vi "LVJSON Unflatten.vi"(7 "Variant Type":variant, 8 "error in (no error)":errorcluster, 10 "Root Path ([]=Root)":string[](array[string]), 11 "Root Element in":T1) -> (0 "error out":errorcluster, 1 "Exists?":bool, 3 "Variant out":variant, 4 "Key":string)   [LabVIEW 2019, in "labview_json.lvlib"]
uses:
  labview_json.lvlib
  Element.ctl
  Element Type.ctl
  <vilib>/Utility/error.llb/Error Cluster From Error Code.vi
  <vilib>/ErrorRing/Error Ring.xnode
  <vilib>/Utility/Data Type/NI_Data Type.lvlib
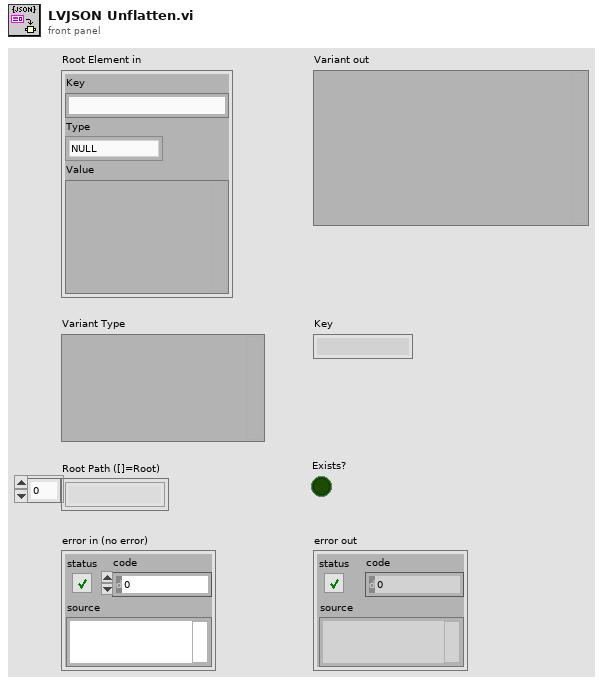
[diagram p1: front panel]
types:
  T1 = typedef "labview_json.lvlib/Element.ctl" = cluster{"Key":string, "Type":T2, "Value":variant}
  T2 = typedef "labview_json.lvlib/Element Type.ctl" = enum8{"NULL", "BOOL", "INT", "UINT", "FLOAT", "STRING", "ARRAY", "OBJECT", "SKIP"}
  T3 = typedef "NI_Data Type.lvlib/Data Type.ctl" = enum8{"Invalid Type", "Void", "I8", "I16", "I32", "I64", "U8", "U16", "U32", "U64", "Single Float", "Double Float", "Extended Float", "Single Complex", "Double Complex", "Extended Complex", "Enum U8", "Enum U16", "Enum U32", "Enum U64", "Single Float With Unit", "Double Float With Unit", "Extended Float With Unit", "Single Complex with Unit", "Double Complex with Unit", "Extended Complex with Unit", "Boolean", "String", "Path", "Picture", "Tag", "Array", "Cluster", "Variant", "LV Variant", "Waveform", "Timestamp", "Digital Waveform", "Digital Data", "ExpressData", "Refnum", "External Data", "VI", "Poly VI", "LabVIEW Class Instance", "Fixed Point", "Set Collection", "Map Collection"}
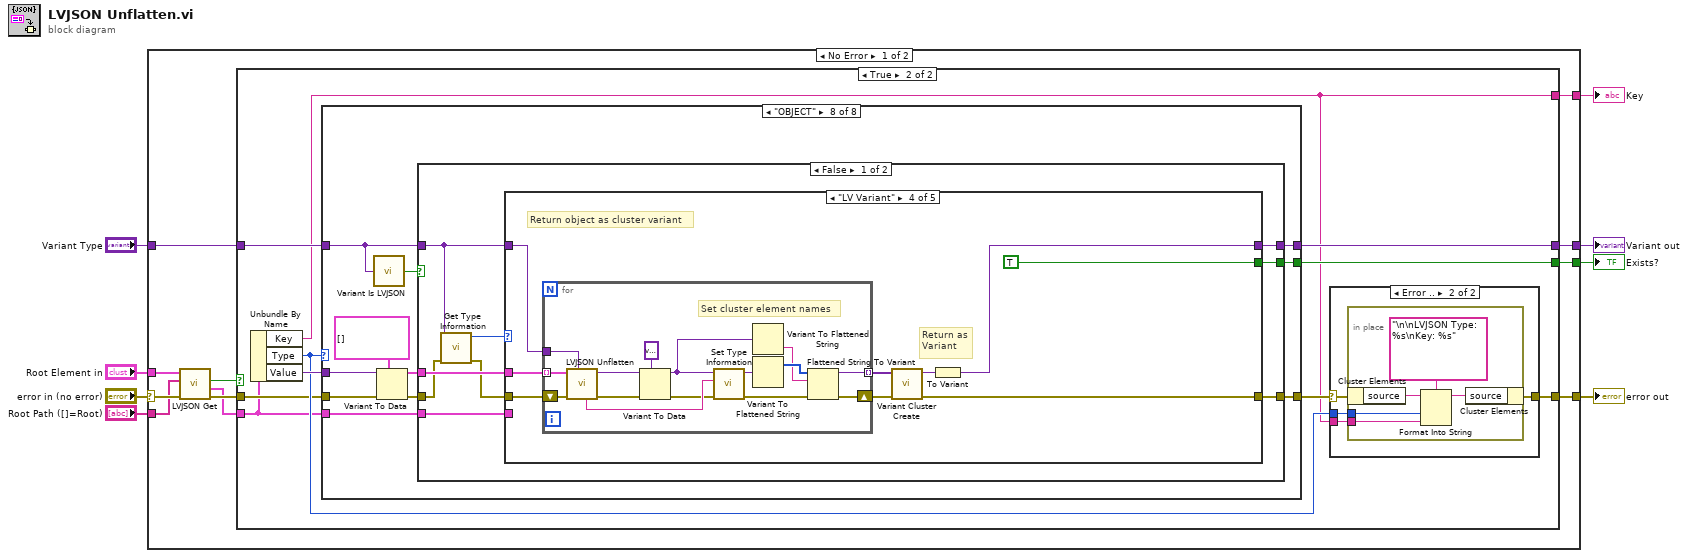
[diagram p0: block diagram]
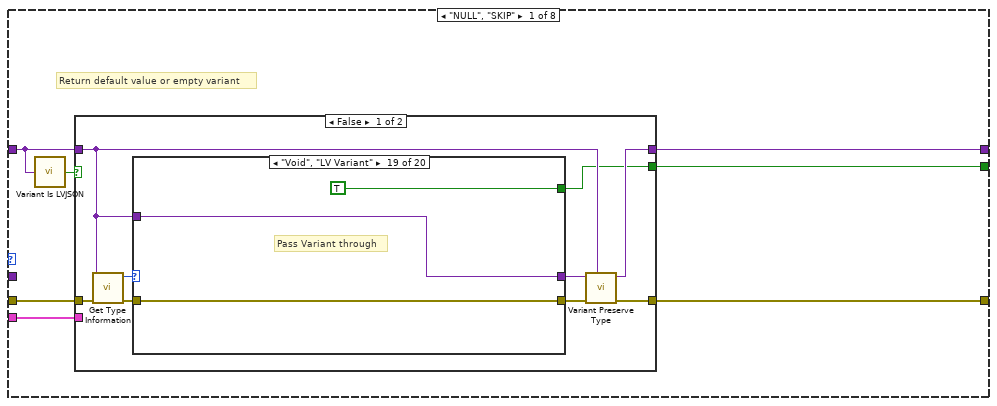
[diagram p3: hidden frame]
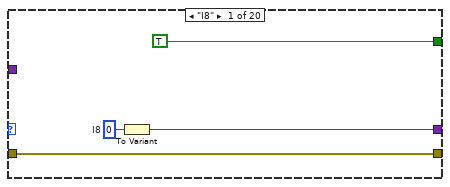
[diagram p4: hidden frame]
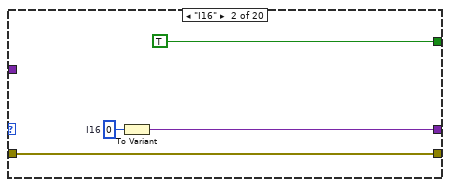
[diagram p5: hidden frame]
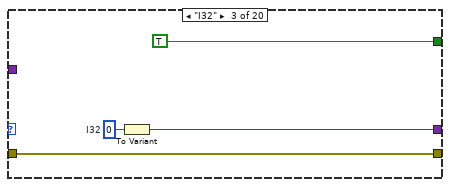
[diagram p6: hidden frame]
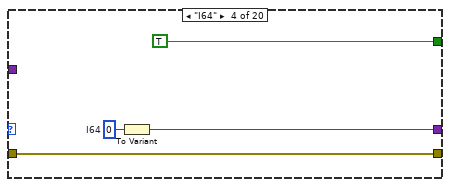
[diagram p7: hidden frame]
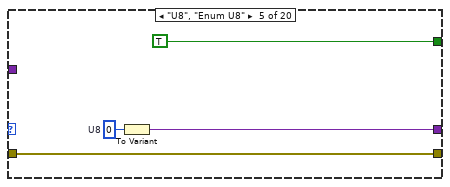
[diagram p8: hidden frame]
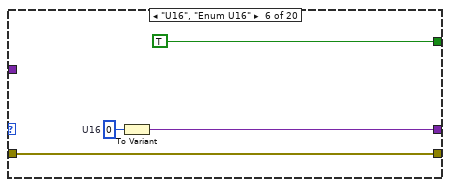
[diagram p9: hidden frame]
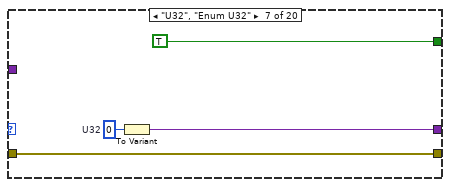
[diagram p10: hidden frame]
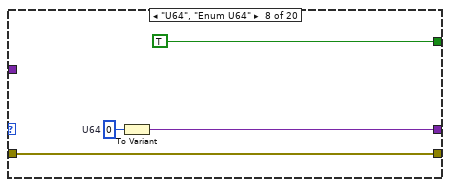
[diagram p11: hidden frame]
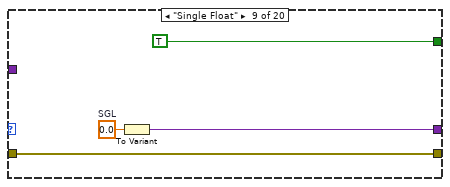
[diagram p12: hidden frame]
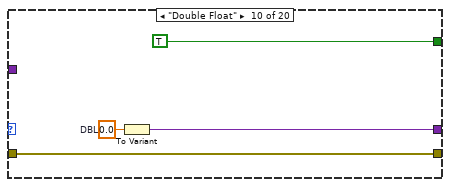
[diagram p13: hidden frame]
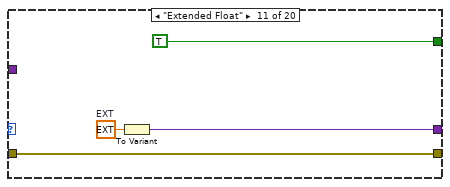
[diagram p14: hidden frame]
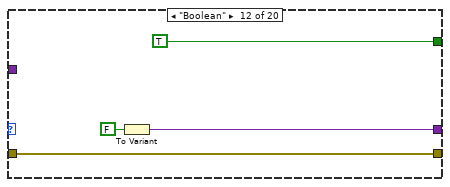
[diagram p15: hidden frame]
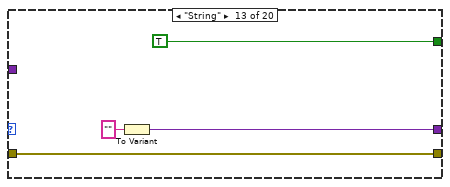
[diagram p16: hidden frame]
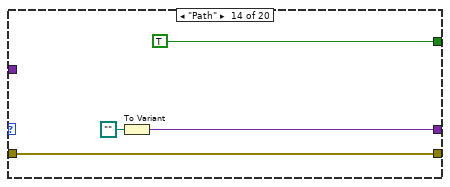
[diagram p17: hidden frame]
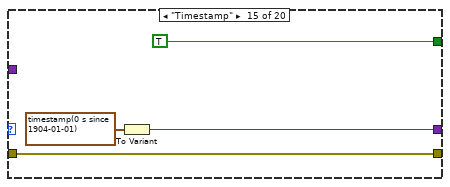
[diagram p18: hidden frame]
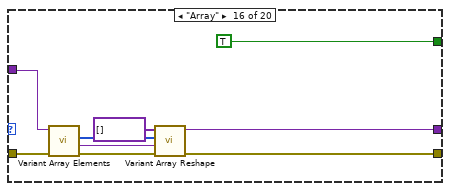
[diagram p19: hidden frame]
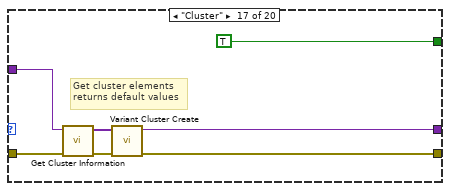
[diagram p20: hidden frame]
diagram:
  n1 = case shown="No Error" "error in (no error)" {
    selector: "error in (no error)" -> [w14 w1004]
    tunnel: "Root Element in" -> [w12 _]
    tunnel: [w19 w1004] -> w8
    tunnel: "Variant Type" -> [w18 w1003]
    tunnel: [w15 _] -> w4
    tunnel: [w17 w1003] -> w3
    tunnel: [w16 _] -> w2
    tunnel: "Root Path ([]=Root)" -> [w11 _]
    frame No Error {
      n2 = call "LVJSON Get.vi"("error in (no error)"=w14, "Root Path ([]=Root)"=w11, "Root Element in"=w12) -> ("error out"=w13:errorcluster, "Element out"=w10:T1, "Exists?"=w9:bool)  [unwired: 5 in, 1 out]
      n3 = case shown="True" w9 {
        tunnel: [w21 w31] -> w19
        tunnel: w18 -> [w20 w30]
        tunnel: [w20 w29] -> w17
        tunnel: [_ w27] -> w16
        tunnel: [_ w24] -> w15
        tunnel: w13 -> [w21 w23]
        tunnel: w10 -> [_ w22]
        frame False {
        }
        frame True {
          n4 = Unbundle By Name(w22) -> ("Key"=w24:string, "Type"=w25:T2, "Value"=w26:variant)
          n5 = case shown="\"OBJECT\"" w25 {
            tunnel: [w38 w160 w213 w317 w421 w525 w664 w834] -> w29
            tunnel: w23 -> [w32 w156 w208 w312 w416 w520 w668 w838]
            tunnel: w30 -> [w35 w150 w205 w309 w413 w517 w661 w830]
            tunnel: w22 -> [w33 w152 w203 w307 w411 w515 w660 w832]
            tunnel: w26 -> [_ w155 w207 w311 w415 w519 w667 w837]
            tunnel: [w37 w159 w212 w316 w420 w524 w663 w833] -> w28
            tunnel: [w36 w154 w206 w310 w414 w518 w662 w831] -> w27
            frame "NULL", "SKIP" {
              # "Return default value or empty variant"
              n6 = call "Variant Is LVJSON.vi"("Variant"=w35) -> ("Is LVJSON?"=w34:bool)
              n7 = case shown="False" w34 {
                tunnel: [w47 w148] -> w38
                tunnel: [w46 w146] -> w37
                tunnel: [w39 TRUE] -> w36
                tunnel: w32 -> [w41 w146]
                tunnel: w35 -> [w40 _]
                tunnel: w33 -> [_ w149]
                frame False {
                  n8 = call <vilib>:"Get Type Information.vi"("error in (no error)"=w41, "variant"=w40) -> ("error out"=w42:errorcluster, "type"=w43:T3)  [unwired: 5 in, 3 out]
                  n9 = case shown="\"Void\", \"LV Variant\"" w43 {
                    selector: w43 -> [_ _ _ _ _ _ _ _ _ _ _ _ _ _ _ _ _ _ _ w133]
                    tunnel: [w51 w55 w59 w63 w67 w71 w75 w79 w83 w87 w91 w95 w99 w103 w107 w112 w122 w127 w130 w132] -> w45
                    tunnel: w42 -> [w51 w55 w59 w63 w67 w71 w75 w79 w83 w87 w91 w95 w99 w103 w107 w110 w121 w127 w130 w137]
                    tunnel: [w50 w54 w58 w62 w66 w70 w74 w78 w82 w86 w90 w94 w98 w102 w106 w111 w118 w126 w128 w138] -> w44
                    tunnel: w40 -> [_ _ _ _ _ _ _ _ _ _ _ _ _ _ _ w109 w120 _ w128 w138]
                    tunnel: [TRUE TRUE TRUE TRUE TRUE TRUE TRUE TRUE TRUE TRUE TRUE TRUE TRUE TRUE TRUE TRUE TRUE TRUE TRUE FALSE] -> w39
                    frame "I8" {
                      w49 = i8 0  # I8
                      n10 = To Variant(anything=w49) -> (Variant=w50:variant)
                    }
                    frame "I16" {
                      w53 = i16 0  # I16
                      n11 = To Variant(anything=w53) -> (Variant=w54:variant)
                    }
                    frame "I32" {
                      w57 = 0  # I32
                      n12 = To Variant(anything=w57) -> (Variant=w58:variant)
                    }
                    frame "I64" {
                      w61 = i64 0  # I64
                      n13 = To Variant(anything=w61) -> (Variant=w62:variant)
                    }
                    frame "U8", "Enum U8" {
                      w65 = u8 0  # U8
                      n14 = To Variant(anything=w65) -> (Variant=w66:variant)
                    }
                    frame "U16", "Enum U16" {
                      w69 = u16 0  # U16
                      n15 = To Variant(anything=w69) -> (Variant=w70:variant)
                    }
                    frame "U32", "Enum U32" {
                      w73 = u32 0  # U32
                      n16 = To Variant(anything=w73) -> (Variant=w74:variant)
                    }
                    frame "U64", "Enum U64" {
                      w77 = u64 0  # U64
                      n17 = To Variant(anything=w77) -> (Variant=w78:variant)
                    }
                    frame "Single Float" {
                      w81 = sgl 0.0  # SGL
                      n18 = To Variant(anything=w81) -> (Variant=w82:variant)
                    }
                    frame "Double Float" {
                      w85 = 0.0  # DBL
                      n19 = To Variant(anything=w85) -> (Variant=w86:variant)
                    }
                    frame "Extended Float" {
                      w89 = ext 0.0  # EXT
                      n20 = To Variant(anything=w89) -> (Variant=w90:variant)
                    }
                    frame "Boolean" {
                      n21 = To Variant(anything=FALSE) -> (Variant=w94:variant)
                    }
                    frame "String" {
                      n22 = To Variant(anything="") -> (Variant=w98:variant)
                    }
                    frame "Path" {
                      n23 = To Variant(anything=path "" ("Not A Path Constant")) -> (Variant=w102:variant)
                    }
                    frame "Timestamp" {
                      n24 = To Variant(anything=timestamp(0 s since 1904-01-01)) -> (Variant=w106:variant)
                    }
                    frame "Array" {
                      n25 = call "Variant Array Elements.vi"("error in (no error)"=w110, "N Dim Array"=w109) -> ("error out"=w113:errorcluster, "Element Type"=w114:variant, "Sizes"=w115:i32[])  [unwired: 6 in, 1 out]
                      n26 = call "Variant Array Reshape.vi"("error in (no error)"=w113, "Default Element Type"=w114, "Sizes"=w115, "Elements"=variant[] []) -> ("error out"=w112:errorcluster, "N Dim Array"=w111:variant)  [unwired: 6 in]
                    }
                    frame "Cluster" {
                      # "Get cluster elements\nreturns default values"
                      n27 = call <vilib>:"Get Cluster Information.vi"("error in (no error)"=w121, "variant"=w120) -> ("error out"=w117:errorcluster, "cluster elements"=w119:variant[])  [unwired: 8 in]
                      n28 = call "Variant Cluster Create.vi"("error in (no error)"=w117, "Elements"=w119) -> ("error out"=w122:errorcluster, "Cluster"=w118:variant)  [unwired: 8 in]
                    }
                    frame "Waveform" {
                      n29 = To Variant(anything=waveform(dbl) {"t0"=timestamp(0 s since 1904-01-01), "dt"=0.0, "Y"=[]} ("Waveform")) -> (Variant=w126:variant)
                    }
                    frame "Void", "LV Variant" {
                      # "Pass Variant through"
                    }
                    frame Default {
                      n30 = Format Into String(format string="%s", w133) -> (resulting string=w135:string)  [unwired: 2 in, 1 out]
                      n31 = xnode "Error Ring"("parameter 0"=w135) -> ("error out"=w131:errorcluster)
                      n32 = Merge Errors(w137, w131) -> (w132:errorcluster)
                    }
                  }
                  n33 = call "Variant Preserve Type.vi"("Variant Type"=w40, "error in (no error)"=w45, "Variant in"=w44) -> ("error out"=w46:errorcluster, "Variant out"=w47:variant)  [unwired: 7 in]
                }
                frame True {
                  # "Return element as LVJSON object"
                  n34 = To Variant(anything=w149) -> (Variant=w148:variant)
                }
              }
            }
            frame "BOOL" {
              # "Return boolean"
              n35 = Variant To Data(error in=w156, type=FALSE, Variant=w155) -> (data=w158:bool, error out=w151:errorcluster)
              n36 = call "Variant Is LVJSON.vi"("Variant"=w150) -> ("Is LVJSON?"=w153:bool)
              n37 = case shown="False" w153 {
                tunnel: [w170 w201] -> w160
                tunnel: [w169 w199] -> w159
                tunnel: w158 -> [w168 _]
                tunnel: [w162 TRUE] -> w154
                tunnel: w151 -> [w165 w199]
                tunnel: w150 -> [w161 _]
                tunnel: w152 -> [_ w202]
                frame False {
                  n38 = call <vilib>:"Get Type Information.vi"("error in (no error)"=w165, "variant"=w161) -> ("error out"=w163:errorcluster, "type"=w166:T3)  [unwired: 5 in, 3 out]
                  n39 = case shown="\"Void\"" w166 {
                    selector: w166 -> [w171 _ _ _]
                    tunnel: w168 -> [_ w189 w193 w197]
                    tunnel: [w177 w188 w191 w195] -> w167
                    tunnel: [w173 w187 w190 w196] -> w164
                    tunnel: w163 -> [w178 w187 w190 w196]
                    tunnel: [FALSE TRUE TRUE TRUE] -> w162
                    tunnel: w161 -> [w177 _ _ _]
                    frame Default {
                      n40 = Format Into String(format string="%s", w171) -> (resulting string=w175:string)  [unwired: 2 in, 1 out]
                      n41 = xnode "Error Ring"("parameter 0"=w175) -> ("error out"=w172:errorcluster)
                      n42 = Merge Errors(w178, w172) -> (w173:errorcluster)
                    }
                    frame "Boolean" {
                      n43 = To Variant(anything=w189) -> (Variant=w188:variant)
                    }
                    frame "LV Variant" {
                      n44 = To Variant(anything=w193) -> (Variant=w192:variant)
                      n45 = To Variant(anything=w192) -> (Variant=w191:variant)
                    }
                    frame "Void" {
                      n46 = To Variant(anything=w197) -> (Variant=w195:variant)
                    }
                  }
                  n47 = call "Variant Preserve Type.vi"("Variant Type"=w161, "error in (no error)"=w164, "Variant in"=w167) -> ("error out"=w169:errorcluster, "Variant out"=w170:variant)  [unwired: 7 in]
                }
                frame True {
                  # "Return element as LVJSON object"
                  n48 = To Variant(anything=w202) -> (Variant=w201:variant)
                }
              }
            }
            frame "INT" {
              w211 = i64 0  # I64
              # "Return int as int, uint, float or variant"
              n49 = call "Variant Is LVJSON.vi"("Variant"=w205) -> ("Is LVJSON?"=w204:bool)
              n50 = Variant To Data(error in=w208, type=w211, Variant=w207) -> (data=w209:i64, error out=w210:errorcluster)
              n51 = case shown="False" w204 {
                tunnel: [w223 w305] -> w213
                tunnel: [w222 w303] -> w212
                tunnel: w210 -> [w217 w303]
                tunnel: w209 -> [w221 _]
                tunnel: [w214 TRUE] -> w206
                tunnel: w205 -> [w215 _]
                tunnel: w203 -> [_ w306]
                frame False {
                  n52 = call <vilib>:"Get Type Information.vi"("error in (no error)"=w217, "variant"=w215) -> ("error out"=w218:errorcluster, "type"=w216:T3)  [unwired: 5 in, 3 out]
                  n53 = case shown="\"Void\"" w216 {
                    selector: w216 -> [w228 _ _ _ _ _ _ _ _ _ _ _ _ _]
                    tunnel: [w227 w242 w247 w252 w257 w262 w267 w272 w277 w282 w287 w292 w298 w302] -> w220
                    tunnel: w218 -> [w231 w242 w247 w252 w257 w262 w267 w272 w277 w282 w287 w292 w298 w302]
                    tunnel: [w225 w240 w245 w250 w255 w260 w265 w270 w275 w280 w285 w290 w296 w299] -> w219
                    tunnel: w221 -> [_ w243 w248 w253 w258 w263 w268 w273 w278 w283 w288 w293 w297 w301]
                    tunnel: w215 -> [w225 _ _ _ _ _ _ _ _ _ _ _ _ _]
                    tunnel: [FALSE TRUE TRUE TRUE TRUE TRUE TRUE TRUE TRUE TRUE TRUE TRUE TRUE TRUE] -> w214
                    frame Default {
                      n54 = Format Into String(format string="%s", w228) -> (resulting string=w230:string)  [unwired: 2 in, 1 out]
                      n55 = xnode "Error Ring"("parameter 0"=w230) -> ("error out"=w226:errorcluster)
                      n56 = Merge Errors(w231, w226) -> (w227:errorcluster)
                    }
                    frame "I8" {
                      n57 = To Byte Integer(number=w243) -> (8bit integer=w241:i8)
                      n58 = To Variant(anything=w241) -> (Variant=w240:variant)
                    }
                    frame "I16" {
                      n59 = To Word Integer(number=w248) -> (16bit integer=w246:i16)
                      n60 = To Variant(anything=w246) -> (Variant=w245:variant)
                    }
                    frame "I32" {
                      n61 = To Long Integer(number=w253) -> (32bit integer=w251:i32)
                      n62 = To Variant(anything=w251) -> (Variant=w250:variant)
                    }
                    frame "I64" {
                      n63 = To Quad Integer(1:w258) -> (0:w256:i64)
                      n64 = To Variant(anything=w256) -> (Variant=w255:variant)
                    }
                    frame "U8", "Enum U8" {
                      n65 = To Unsigned Byte Integer(number=w263) -> (unsigned 8bit integer=w261:u8)
                      n66 = To Variant(anything=w261) -> (Variant=w260:variant)
                    }
                    frame "U16", "Enum U16" {
                      n67 = To Unsigned Word Integer(number=w268) -> (unsigned 16bit integer=w266:u16)
                      n68 = To Variant(anything=w266) -> (Variant=w265:variant)
                    }
                    frame "U32", "Enum U32" {
                      n69 = To Unsigned Long Integer(number=w273) -> (unsigned 32bit integer=w271:u32)
                      n70 = To Variant(anything=w271) -> (Variant=w270:variant)
                    }
                    frame "U64", "Enum U64" {
                      n71 = To Unsigned Quad Integer(1:w278) -> (0:w276:u64)
                      n72 = To Variant(anything=w276) -> (Variant=w275:variant)
                    }
                    frame "Single Float" {
                      n73 = To Single Precision Float(number=w283) -> (single precision float=w281:sgl)
                      n74 = To Variant(anything=w281) -> (Variant=w280:variant)
                    }
                    frame "Double Float" {
                      n75 = To Double Precision Float(number=w288) -> (double precision float=w286:dbl)
                      n76 = To Variant(anything=w286) -> (Variant=w285:variant)
                    }
                    frame "Extended Float" {
                      n77 = To Extended Precision Float(1:w293) -> (0:w291:ext)
                      n78 = To Variant(anything=w291) -> (Variant=w290:variant)
                    }
                    frame "LV Variant" {
                      n79 = To Variant(anything=w297) -> (Variant=w295:variant)
                      n80 = To Variant(anything=w295) -> (Variant=w296:variant)
                    }
                    frame "Void" {
                      n81 = To Variant(anything=w301) -> (Variant=w299:variant)
                    }
                  }
                  n82 = call "Variant Preserve Type.vi"("Variant Type"=w215, "error in (no error)"=w220, "Variant in"=w219) -> ("error out"=w222:errorcluster, "Variant out"=w223:variant)  [unwired: 7 in]
                }
                frame True {
                  # "Return element as LVJSON object"
                  n83 = To Variant(anything=w306) -> (Variant=w305:variant)
                }
              }
            }
            frame "UINT" {
              w315 = u64 0  # U64
              # "Return int as int, uint, float or variant"
              n84 = call "Variant Is LVJSON.vi"("Variant"=w309) -> ("Is LVJSON?"=w308:bool)
              n85 = Variant To Data(error in=w312, type=w315, Variant=w311) -> (data=w313:u64, error out=w314:errorcluster)
              n86 = case shown="False" w308 {
                tunnel: [w327 w409] -> w317
                tunnel: [w326 w407] -> w316
                tunnel: w314 -> [w321 w407]
                tunnel: w313 -> [w325 _]
                tunnel: [w318 TRUE] -> w310
                tunnel: w309 -> [w319 _]
                tunnel: w307 -> [_ w410]
                frame False {
                  n87 = call <vilib>:"Get Type Information.vi"("error in (no error)"=w321, "variant"=w319) -> ("error out"=w322:errorcluster, "type"=w320:T3)  [unwired: 5 in, 3 out]
                  n88 = case shown="\"Void\"" w320 {
                    selector: w320 -> [w332 _ _ _ _ _ _ _ _ _ _ _ _ _]
                    tunnel: [w331 w346 w351 w356 w361 w366 w371 w376 w381 w386 w391 w396 w402 w406] -> w324
                    tunnel: w322 -> [w335 w346 w351 w356 w361 w366 w371 w376 w381 w386 w391 w396 w402 w406]
                    tunnel: [w329 w344 w349 w354 w359 w364 w369 w374 w379 w384 w389 w394 w400 w403] -> w323
                    tunnel: w325 -> [_ w347 w352 w357 w362 w367 w372 w377 w382 w387 w392 w397 w401 w405]
                    tunnel: w319 -> [w329 _ _ _ _ _ _ _ _ _ _ _ _ _]
                    tunnel: [FALSE TRUE TRUE TRUE TRUE TRUE TRUE TRUE TRUE TRUE TRUE TRUE TRUE TRUE] -> w318
                    frame Default {
                      n89 = Format Into String(format string="%s", w332) -> (resulting string=w334:string)  [unwired: 2 in, 1 out]
                      n90 = xnode "Error Ring"("parameter 0"=w334) -> ("error out"=w330:errorcluster)
                      n91 = Merge Errors(w335, w330) -> (w331:errorcluster)
                    }
                    frame "I8" {
                      n92 = To Byte Integer(number=w347) -> (8bit integer=w345:i8)
                      n93 = To Variant(anything=w345) -> (Variant=w344:variant)
                    }
                    frame "I16" {
                      n94 = To Word Integer(number=w352) -> (16bit integer=w350:i16)
                      n95 = To Variant(anything=w350) -> (Variant=w349:variant)
                    }
                    frame "I32" {
                      n96 = To Long Integer(number=w357) -> (32bit integer=w355:i32)
                      n97 = To Variant(anything=w355) -> (Variant=w354:variant)
                    }
                    frame "I64" {
                      n98 = To Quad Integer(1:w362) -> (0:w360:i64)
                      n99 = To Variant(anything=w360) -> (Variant=w359:variant)
                    }
                    frame "U8", "Enum U8" {
                      n100 = To Unsigned Byte Integer(number=w367) -> (unsigned 8bit integer=w365:u8)
                      n101 = To Variant(anything=w365) -> (Variant=w364:variant)
                    }
                    frame "U16", "Enum U16" {
                      n102 = To Unsigned Word Integer(number=w372) -> (unsigned 16bit integer=w370:u16)
                      n103 = To Variant(anything=w370) -> (Variant=w369:variant)
                    }
                    frame "U32", "Enum U32" {
                      n104 = To Unsigned Long Integer(number=w377) -> (unsigned 32bit integer=w375:u32)
                      n105 = To Variant(anything=w375) -> (Variant=w374:variant)
                    }
                    frame "U64", "Enum U64" {
                      n106 = To Unsigned Quad Integer(1:w382) -> (0:w380:u64)
                      n107 = To Variant(anything=w380) -> (Variant=w379:variant)
                    }
                    frame "Single Float" {
                      n108 = To Single Precision Float(number=w387) -> (single precision float=w385:sgl)
                      n109 = To Variant(anything=w385) -> (Variant=w384:variant)
                    }
                    frame "Double Float" {
                      n110 = To Double Precision Float(number=w392) -> (double precision float=w390:dbl)
                      n111 = To Variant(anything=w390) -> (Variant=w389:variant)
                    }
                    frame "Extended Float" {
                      n112 = To Extended Precision Float(1:w397) -> (0:w395:ext)
                      n113 = To Variant(anything=w395) -> (Variant=w394:variant)
                    }
                    frame "LV Variant" {
                      n114 = To Variant(anything=w401) -> (Variant=w399:variant)
                      n115 = To Variant(anything=w399) -> (Variant=w400:variant)
                    }
                    frame "Void" {
                      n116 = To Variant(anything=w405) -> (Variant=w403:variant)
                    }
                  }
                  n117 = call "Variant Preserve Type.vi"("Variant Type"=w319, "error in (no error)"=w324, "Variant in"=w323) -> ("error out"=w326:errorcluster, "Variant out"=w327:variant)  [unwired: 7 in]
                }
                frame True {
                  # "Return element as LVJSON object"
                  n118 = To Variant(anything=w410) -> (Variant=w409:variant)
                }
              }
            }
            frame "FLOAT" {
              w419 = 0.0  # DBL
              # "Return int as int, uint, float or variant"
              n119 = call "Variant Is LVJSON.vi"("Variant"=w413) -> ("Is LVJSON?"=w412:bool)
              n120 = Variant To Data(error in=w416, type=w419, Variant=w415) -> (data=w417:dbl, error out=w418:errorcluster)
              n121 = case shown="False" w412 {
                tunnel: [w431 w513] -> w421
                tunnel: [w430 w511] -> w420
                tunnel: w418 -> [w425 w511]
                tunnel: w417 -> [w429 _]
                tunnel: [w422 TRUE] -> w414
                tunnel: w413 -> [w423 _]
                tunnel: w411 -> [_ w514]
                frame False {
                  n122 = call <vilib>:"Get Type Information.vi"("error in (no error)"=w425, "variant"=w423) -> ("error out"=w426:errorcluster, "type"=w424:T3)  [unwired: 5 in, 3 out]
                  n123 = case shown="\"Void\"" w424 {
                    selector: w424 -> [w436 _ _ _ _ _ _ _ _ _ _ _ _ _]
                    tunnel: [w435 w450 w455 w460 w465 w470 w475 w480 w485 w490 w495 w500 w506 w510] -> w428
                    tunnel: w426 -> [w439 w450 w455 w460 w465 w470 w475 w480 w485 w490 w495 w500 w506 w510]
                    tunnel: [w433 w448 w453 w458 w463 w468 w473 w478 w483 w488 w493 w498 w504 w507] -> w427
                    tunnel: w429 -> [_ w451 w456 w461 w466 w471 w476 w481 w486 w491 w496 w501 w505 w509]
                    tunnel: w423 -> [w433 _ _ _ _ _ _ _ _ _ _ _ _ _]
                    tunnel: [FALSE TRUE TRUE TRUE TRUE TRUE TRUE TRUE TRUE TRUE TRUE TRUE TRUE TRUE] -> w422
                    frame Default {
                      n124 = Format Into String(format string="%s", w436) -> (resulting string=w438:string)  [unwired: 2 in, 1 out]
                      n125 = xnode "Error Ring"("parameter 0"=w438) -> ("error out"=w434:errorcluster)
                      n126 = Merge Errors(w439, w434) -> (w435:errorcluster)
                    }
                    frame "I8" {
                      n127 = To Byte Integer(number=w451) -> (8bit integer=w449:i8)
                      n128 = To Variant(anything=w449) -> (Variant=w448:variant)
                    }
                    frame "I16" {
                      n129 = To Word Integer(number=w456) -> (16bit integer=w454:i16)
                      n130 = To Variant(anything=w454) -> (Variant=w453:variant)
                    }
                    frame "I32" {
                      n131 = To Long Integer(number=w461) -> (32bit integer=w459:i32)
                      n132 = To Variant(anything=w459) -> (Variant=w458:variant)
                    }
                    frame "I64" {
                      n133 = To Quad Integer(1:w466) -> (0:w464:i64)
                      n134 = To Variant(anything=w464) -> (Variant=w463:variant)
                    }
                    frame "U8", "Enum U8" {
                      n135 = To Unsigned Byte Integer(number=w471) -> (unsigned 8bit integer=w469:u8)
                      n136 = To Variant(anything=w469) -> (Variant=w468:variant)
                    }
                    frame "U16", "Enum U16" {
                      n137 = To Unsigned Word Integer(number=w476) -> (unsigned 16bit integer=w474:u16)
                      n138 = To Variant(anything=w474) -> (Variant=w473:variant)
                    }
                    frame "U32", "Enum U32" {
                      n139 = To Unsigned Long Integer(number=w481) -> (unsigned 32bit integer=w479:u32)
                      n140 = To Variant(anything=w479) -> (Variant=w478:variant)
                    }
                    frame "U64", "Enum U64" {
                      n141 = To Unsigned Quad Integer(1:w486) -> (0:w484:u64)
                      n142 = To Variant(anything=w484) -> (Variant=w483:variant)
                    }
                    frame "Single Float" {
                      n143 = To Single Precision Float(number=w491) -> (single precision float=w489:sgl)
                      n144 = To Variant(anything=w489) -> (Variant=w488:variant)
                    }
                    frame "Double Float" {
                      n145 = To Double Precision Float(number=w496) -> (double precision float=w494:dbl)
                      n146 = To Variant(anything=w494) -> (Variant=w493:variant)
                    }
                    frame "Extended Float" {
                      n147 = To Extended Precision Float(1:w501) -> (0:w499:ext)
                      n148 = To Variant(anything=w499) -> (Variant=w498:variant)
                    }
                    frame "LV Variant" {
                      n149 = To Variant(anything=w505) -> (Variant=w503:variant)
                      n150 = To Variant(anything=w503) -> (Variant=w504:variant)
                    }
                    frame "Void" {
                      n151 = To Variant(anything=w509) -> (Variant=w507:variant)
                    }
                  }
                  n152 = call "Variant Preserve Type.vi"("Variant Type"=w423, "error in (no error)"=w428, "Variant in"=w427) -> ("error out"=w430:errorcluster, "Variant out"=w431:variant)  [unwired: 7 in]
                }
                frame True {
                  # "Return element as LVJSON object"
                  n153 = To Variant(anything=w514) -> (Variant=w513:variant)
                }
              }
            }
            frame "STRING" {
              # "Return string as string, enum, path, timestamp or variant"
              n154 = Variant To Data(error in=w520, type="", Variant=w519) -> (data=w522:string, error out=w523:errorcluster)
              n155 = call "Variant Is LVJSON.vi"("Variant"=w517) -> ("Is LVJSON?"=w516:bool)
              n156 = case shown="False" w516 {
                tunnel: [w535 w657] -> w525
                tunnel: [w534 w655] -> w524
                tunnel: w523 -> [w528 w655]
                tunnel: w522 -> [w533 _]
                tunnel: w517 -> [w530 _]
                tunnel: [w526 TRUE] -> w518
                tunnel: w515 -> [_ w658]
                frame False {
                  n157 = call <vilib>:"Get Type Information.vi"("error in (no error)"=w528, "variant"=w530) -> ("error out"=w529:errorcluster, "type"=w527:T3)  [unwired: 5 in, 3 out]
                  n158 = case shown="\"Void\"" w527 {
                    selector: w527 -> [w538 _ _ _ _ _ _ _ _]
                    tunnel: [w537 w553 w580 w607 w635 w640 w645 w649 w654] -> w531
                    tunnel: w529 -> [w543 w557 w584 w611 w635 w640 w645 w649 w654]
                    tunnel: [w542 w560 w587 w614 w634 w639 w643 w646 w653] -> w532
                    tunnel: w533 -> [_ w556 w583 w610 w633 w638 w644 w648 w652]
                    tunnel: w530 -> [w542 w559 w586 w613 _ _ _ _ _]
                    tunnel: [FALSE w552 w579 w606 TRUE TRUE TRUE TRUE TRUE] -> w526
                    frame Default {
                      n159 = Format Into String(format string="%s", w538) -> (resulting string=w540:string)  [unwired: 2 in, 1 out]
                      n160 = xnode "Error Ring"("parameter 0"=w540) -> ("error out"=w536:errorcluster)
                      n161 = Merge Errors(w543, w536) -> (w537:errorcluster)
                    }
                    frame "Enum U8" {
                      n162 = call <vilib>:"Get Numeric Information.vi"("error in (no error)"=w557, "variant"=w559) -> ("error out"=w554:errorcluster, "enum names"=w558:string[])  [unwired: 6 in, 2 out]
                      n163 = Search 1D Array(1D array=w558, element=w556) -> (index of element=w555:i32)  [unwired: 1 in]
                      n164 = case shown="..-1" w555 {
                        selector: w555 -> [w562 _]
                        tunnel: w556 -> [_ w570]
                        tunnel: w554 -> [w563 w569]
                        tunnel: [w563 w566] -> w553
                        tunnel: [TRUE FALSE] -> w552
                        tunnel: [w564 u8 0] -> w551
                        frame 0.. {
                          n165 = To Unsigned Byte Integer(number=w562) -> (unsigned 8bit integer=w564:u8)
                        }
                        frame ..-1 {
                          n166 = xnode "Error Ring"("parameter 0"=w570) -> ("error out"=w565:errorcluster)
                          n167 = Merge Errors(w569, w565) -> (w566:errorcluster)
                        }
                      }
                      n168 = To Variant(anything=w551) -> (Variant=w560:variant)
                    }
                    frame "Enum U16" {
                      n169 = call <vilib>:"Get Numeric Information.vi"("error in (no error)"=w584, "variant"=w586) -> ("error out"=w581:errorcluster, "enum names"=w585:string[])  [unwired: 6 in, 2 out]
                      n170 = Search 1D Array(1D array=w585, element=w583) -> (index of element=w582:i32)  [unwired: 1 in]
                      n171 = case shown="..-1" w582 {
                        selector: w582 -> [w589 _]
                        tunnel: w583 -> [_ w597]
                        tunnel: w581 -> [w590 w596]
                        tunnel: [w590 w593] -> w580
                        tunnel: [TRUE FALSE] -> w579
                        tunnel: [w591 u16 0] -> w578
                        frame 0.. {
                          n172 = To Unsigned Word Integer(number=w589) -> (unsigned 16bit integer=w591:u16)
                        }
                        frame ..-1 {
                          n173 = xnode "Error Ring"("parameter 0"=w597) -> ("error out"=w592:errorcluster)
                          n174 = Merge Errors(w596, w592) -> (w593:errorcluster)
                        }
                      }
                      n175 = To Variant(anything=w578) -> (Variant=w587:variant)
                    }
                    frame "Enum U32" {
                      n176 = call <vilib>:"Get Numeric Information.vi"("error in (no error)"=w611, "variant"=w613) -> ("error out"=w608:errorcluster, "enum names"=w612:string[])  [unwired: 6 in, 2 out]
                      n177 = Search 1D Array(1D array=w612, element=w610) -> (index of element=w609:i32)  [unwired: 1 in]
                      n178 = case shown="..-1" w609 {
                        selector: w609 -> [w616 _]
                        tunnel: w610 -> [_ w624]
                        tunnel: w608 -> [w617 w623]
                        tunnel: [w617 w620] -> w607
                        tunnel: [TRUE FALSE] -> w606
                        tunnel: [w618 u32 0] -> w605
                        frame 0.. {
                          n179 = To Unsigned Long Integer(number=w616) -> (unsigned 32bit integer=w618:u32)
                        }
                        frame ..-1 {
                          n180 = xnode "Error Ring"("parameter 0"=w624) -> ("error out"=w619:errorcluster)
                          n181 = Merge Errors(w623, w619) -> (w620:errorcluster)
                        }
                      }
                      n182 = To Variant(anything=w605) -> (Variant=w614:variant)
                    }
                    frame "String" {
                      n183 = To Variant(anything=w633) -> (Variant=w634:variant)
                    }
                    frame "Path" {
                      n184 = String To Path(string=w638) -> (path=w637:path)
                      n185 = To Variant(anything=w637) -> (Variant=w639:variant)
                    }
                    frame "LV Variant" {
                      n186 = To Variant(anything=w644) -> (Variant=w642:variant)
                      n187 = To Variant(anything=w642) -> (Variant=w643:variant)
                    }
                    frame "Void" {
                      n188 = To Variant(anything=w648) -> (Variant=w646:variant)
                    }
                    frame "Timestamp" {
                      n189 = call "JSON ISO8601 to Timestamp.vi"("ISO 8601 Date Time"=w652) -> ("Local Time Stamp"=w651:timestamp)  [unwired: 10 in]
                      n190 = To Variant(anything=w651) -> (Variant=w653:variant)
                    }
                  }
                  n191 = call "Variant Preserve Type.vi"("Variant Type"=w530, "error in (no error)"=w531, "Variant in"=w532) -> ("error out"=w534:errorcluster, "Variant out"=w535:variant)  [unwired: 7 in]
                }
                frame True {
                  # "Return element as LVJSON object"
                  n192 = To Variant(anything=w658) -> (Variant=w657:variant)
                }
              }
            }
            frame "ARRAY" {
              n193 = call "Variant Is LVJSON.vi"("Variant"=w661) -> ("Is LVJSON?"=w659:bool)
              n194 = Variant To Data(error in=w668, type=T1[] [], Variant=w667) -> (data=w665:T1[], error out=w666:errorcluster)
              n195 = case shown="False" w659 {
                tunnel: w666 -> [w672 w825]
                tunnel: w665 -> [w677 _]
                tunnel: [w676 w827] -> w664
                tunnel: [w675 w825] -> w663
                tunnel: [w674 TRUE] -> w662
                tunnel: w661 -> [w671 _]
                tunnel: w660 -> [_ w828]
                frame False {
                  n196 = call <vilib>:"Get Type Information.vi"("error in (no error)"=w672, "variant"=w671) -> ("error out"=w673:errorcluster, "type"=w670:T3)  [unwired: 5 in, 3 out]
                  n197 = case shown="\"Void\"" w670 {
                    selector: w670 -> [w679 _ _ _]
                    tunnel: [w683 w698 w798 w816] -> w675
                    tunnel: w673 -> [w684 w701 w800 w818]
                    tunnel: w677 -> [_ w697 w802 w819]
                    tunnel: w671 -> [w685 w695 w790 w813]
                    tunnel: [w685 w694 w797 w815] -> w676
                    tunnel: [FALSE w693 TRUE TRUE] -> w674
                    frame Default {
                      n198 = Format Into String(format string="%s", w679) -> (resulting string=w682:string)  [unwired: 2 in, 1 out]
                      n199 = xnode "Error Ring"("parameter 0"=w682) -> ("error out"=w680:errorcluster)
                      n200 = Merge Errors(w684, w680) -> (w683:errorcluster)
                    }
                    frame "Array" {
                      # "Return array"
                      n201 = call <vilib>:"Get Array Information.vi"("error in (no error)"=w701, "variant"=w695) -> ("error out"=w699:errorcluster, "array element data type"=w696:variant, "number of dimensions"=w700:i32)  [unwired: 6 in, 1 out]
                      n202 = case shown="2.." w700 {
                        selector: w700 -> [w703 _ _]
                        tunnel: w699 -> [w705 w716 w757]
                        tunnel: [w704 w730 w762] -> w698
                        tunnel: w697 -> [_ w722 w755]
                        tunnel: w696 -> [_ w724 _]
                        tunnel: [w707 w728 w761] -> w694
                        tunnel: w695 -> [w707 w727 w756]
                        tunnel: [FALSE w725 w760] -> w693
                        frame ..0 {
                          n203 = xnode "Error Ring"("parameter 0"=w703) -> ("error out"=w706:errorcluster)
                          n204 = Merge Errors(w705, w706) -> (w704:errorcluster)
                        }
                        frame 1 {
                          # "Keep existing elements in array"
                          n205 = Array Size(array=w722) -> (size(s)=w721:i32)
                          n206 = Initialize Array(w724, w721) -> (w720:variant[])
                          n207 = Variant To Data(error in=w716, type=variant[] [], Variant=w727) -> (data=w719:variant[], error out=w715:errorcluster)
                          n208 = Replace Array Subset(array=w720, new element=w719, index=0) -> (w717:variant[])
                          n209 = for {
                            tunnel: w722 -> [w752] mode=indexing
                            shift-right: [w751] -> w734
                            shift-left: w715 -> [w753]
                            tunnel: [w750] -> w733 mode=indexing
                            tunnel: [w746] -> w726 mode=indexing
                            tunnel: w717 -> [w744]
                            i -> [w745]
                            n210 = Index Array(array=w744, index=w745) -> (element=w743:variant)
                            n211 = call "LVJSON Unflatten.vi"("Variant Type"=w743, "error in (no error)"=w753, "Root Element in"=w752) -> ("error out"=w748:errorcluster, "Exists?"=w746:bool, "Variant out"=w747:variant)  [unwired: 5 in, 1 out]
                            n212 = Variant To Data(error in=w748, type=variant, Variant=w747) -> (data=w750:variant, error out=w751:errorcluster)
                          }
                          n213 = And Array Elements(Boolean array=w726) -> (logical AND=w725:bool)
                          n214 = call <vilib>:"Get Type Information.vi"("variant"=w724) -> ("type"=w723:T3)  [unwired: 6 in, 4 out]
                          n215 = case shown="Default" w723 {
                            tunnel: w734 -> [w735 w742]
                            tunnel: w733 -> [w737 w741]
                            tunnel: [w736 w740] -> w729
                            tunnel: [w735 w739] -> w731
                            tunnel: w724 -> [_ w738]
                            frame "LV Variant" {
                              n216 = To Variant(anything=w737) -> (Variant=w736:variant)
                            }
                            frame Default {
                              n217 = call "Variant Array Create.vi"("error in (no error)"=w742, "Default Element Type (if empty)"=w738, "Elements"=w741) -> ("error out"=w739:errorcluster, "Array"=w740:variant)  [unwired: 7 in]
                            }
                          }
                          n218 = call "Variant Preserve Type.vi"("Variant Type"=w727, "error in (no error)"=w731, "Variant in"=w729) -> ("error out"=w730:errorcluster, "Variant out"=w728:variant)  [unwired: 7 in]
                        }
                        frame 2.. {
                          # "Convert to 1d array of variant arrays"
                          n219 = Empty Array?(array=w755) -> (empty?=w754:bool)
                          n220 = case shown="False" w754 {
                            tunnel: w755 -> [w774 _]
                            tunnel: [w772 TRUE] -> w760
                            tunnel: [w770 w783] -> w759
                            tunnel: [w769 w782] -> w758
                            tunnel: w757 -> [w767 w785]
                            tunnel: w756 -> [w766 w784]
                            frame False {
                              n221 = call "Variant Array Decimate.vi"("error in (no error)"=w767, "N Dim Array"=w766) -> ("error out"=w765:errorcluster, "Variant Array Type"=w763:variant, "Element Type"=w764:variant)  [unwired: 6 in, 1 out]
                              n222 = for {
                                shift-right: [w776] -> w771
                                shift-left: w765 -> [w780]
                                tunnel: w774 -> [w778] mode=indexing
                                tunnel: [w779] -> w773 mode=indexing
                                tunnel: [w777] -> w768 mode=indexing
                                tunnel: w763 -> [w775]
                                n223 = call "LVJSON Unflatten.vi"("Variant Type"=w775, "error in (no error)"=w780, "Root Element in"=w778) -> ("error out"=w776:errorcluster, "Exists?"=w779:bool, "Variant out"=w777:variant)  [unwired: 5 in, 1 out]
                              }
                              n224 = And Array Elements(Boolean array=w773) -> (logical AND=w772:bool)
                              n225 = call "Variant Array Interleave.vi"("error in (no error)"=w771, "Default Element Type"=w764, "Array of Variant Arrays"=w768) -> ("error out"=w770:errorcluster, "N Dim Array out"=w769:variant)  [unwired: 7 in]
                            }
                            frame True {
                              # "Empty array"
                              n226 = call "Variant Array Elements.vi"("error in (no error)"=w785, "N Dim Array"=w784) -> ("error out"=w787:errorcluster, "Element Type"=w788:variant, "Sizes"=w789:i32[])  [unwired: 6 in, 1 out]
                              n227 = call "Variant Array Reshape.vi"("error in (no error)"=w787, "Default Element Type"=w788, "Sizes"=w789, "Elements"=variant[] []) -> ("error out"=w783:errorcluster, "N Dim Array"=w782:variant)  [unwired: 6 in]
                            }
                          }
                          n228 = call "Variant Preserve Type.vi"("Variant Type"=w756, "error in (no error)"=w759, "Variant in"=w758) -> ("error out"=w762:errorcluster, "Variant out"=w761:variant)  [unwired: 7 in]
                        }
                      }
                    }
                    frame "LV Variant" {
                      # "Remove\nlabel"
                      # "LV Variant"
                      # "Array of\nVariants"
                      # "Return array as variant"
                      n229 = for {
                        tunnel: w802 -> [w809] mode=indexing
                        shift-right: [w805] -> w794
                        shift-left: w800 -> [w810]
                        tunnel: [w804] -> w799 mode=indexing
                        tunnel: w790 -> [w803]
                        n230 = call "LVJSON Unflatten.vi"("Variant Type"=w803, "error in (no error)"=w810, "Root Element in"=w809) -> ("error out"=w807:errorcluster, "Variant out"=w806:variant)  [unwired: 5 in, 2 out]
                        n231 = Variant To Data(error in=w807, type=variant, Variant=w806) -> (data=w804:variant, error out=w805:errorcluster)
                      }
                      n232 = To Variant(anything=w799) -> (Variant=w801:variant)
                      n233 = To Variant(anything=w801) -> (Variant=w795:variant)
                      n234 = Variant To Data(error in=w794, type=variant, Variant=w795) -> (data=w792:variant, error out=w793:errorcluster)
                      n235 = call "Variant Preserve Type.vi"("Variant Type"=w790, "error in (no error)"=w793, "Variant in"=w792) -> ("error out"=w798:errorcluster, "Variant out"=w797:variant)  [unwired: 7 in]
                    }
                    frame "Void" {
                      # "Array of\nVariants"
                      # "Return array as variant"
                      n236 = for {
                        tunnel: w819 -> [w823] mode=indexing
                        shift-right: [w820] -> w811
                        shift-left: w818 -> [w824]
                        tunnel: [w821] -> w817 mode=indexing
                        tunnel: w813 -> [w822]
                        n237 = call "LVJSON Unflatten.vi"("Variant Type"=w822, "error in (no error)"=w824, "Root Element in"=w823) -> ("error out"=w820:errorcluster, "Variant out"=w821:variant)  [unwired: 5 in, 2 out]
                      }
                      n238 = To Variant(anything=w817) -> (Variant=w812:variant)
                      n239 = call "Variant Preserve Type.vi"("Variant Type"=w813, "error in (no error)"=w811, "Variant in"=w812) -> ("error out"=w816:errorcluster, "Variant out"=w815:variant)  [unwired: 7 in]
                    }
                  }
                }
                frame True {
                  # "Return element as LVJSON object"
                  n240 = To Variant(anything=w828) -> (Variant=w827:variant)
                }
              }
            }
            frame "OBJECT" {
              n241 = call "Variant Is LVJSON.vi"("Variant"=w830) -> ("Is LVJSON?"=w829:bool)
              n242 = Variant To Data(error in=w838, type=T1[] [], Variant=w837) -> (data=w835:T1[], error out=w836:errorcluster)
              n243 = case shown="False" w829 {
                tunnel: w836 -> [w842 w989]
                tunnel: w835 -> [w848 _]
                tunnel: [w847 w991] -> w834
                tunnel: [w846 w989] -> w833
                tunnel: w832 -> [w845 w992]
                tunnel: [w844 TRUE ("Exists?")] -> w831
                tunnel: w830 -> [w841 _]
                frame False {
                  n244 = call <vilib>:"Get Type Information.vi"("error in (no error)"=w842, "variant"=w841) -> ("error out"=w843:errorcluster, "type"=w840:T3)  [unwired: 5 in, 3 out]
                  n245 = case shown="\"LV Variant\"" w840 {
                    selector: w840 -> [w852 _ _ _ _]
                    tunnel: [w853 w878 w944 w951 w974] -> w846
                    tunnel: w843 -> [w854 w874 w927 w947 w972]
                    tunnel: w848 -> [_ w873 _ w946 w971]
                    tunnel: w841 -> [w856 w875 w926 w945 w970]
                    tunnel: [w856 w877 w943 w949 w969] -> w847
                    tunnel: w845 -> [_ _ w923 _ _]
                    tunnel: [FALSE ("Exists?") w865 w922 TRUE ("Exists?") TRUE ("Exists?")] -> w844
                    frame Default {
                      n246 = Format Into String(format string="%s", w852) -> (resulting string=w851:string)  [unwired: 2 in, 1 out]
                      n247 = xnode "Error Ring"("parameter 0"=w851) -> ("error out"=w855:errorcluster)
                      n248 = Merge Errors(w854, w855) -> (w853:errorcluster)
                    }
                    frame "Cluster" {
                      # "Is NULL variant?"
                      # "Return cluster"
                      n249 = Variant To Data(error in=w874, type=variant[] [], Variant=w875) -> (data=w869:variant[], error out=w872:errorcluster)
                      n250 = Array Size(array=w869) -> (size(s)=w871:i32)
                      n251 = Index Array(array=w869) -> (element=w868:variant)  [unwired: 1 in]
                      n252 = Equal?(x=w871, y=1) -> (x = y?=w866:bool)
                      n253 = Empty String/Path?(string/path=w868) -> (empty?=w867:bool)
                      n254 = And(x=w866, y=w867) -> (x .and. y?=w864:bool)
                      n255 = case shown="False" w864 {
                        tunnel: [w891 w918] -> w878
                        tunnel: [w890 w920] -> w877
                        tunnel: w875 -> [w889 w920]
                        tunnel: w873 -> [w888 _]
                        tunnel: w872 -> [w887 w918]
                        tunnel: w871 -> [w886 _]
                        tunnel: w869 -> [w885 _]
                        tunnel: [w884 TRUE] -> w865
                        frame False {
                          n256 = for {
                            N: w886 -> [_]
                            shift-right: [w893] -> w883
                            shift-left: w887 -> [w894]
                            shift-right: [w896] -> w881
                            shift-left: w885 -> [w898]
                            tunnel: w888 -> [w895]
                            tunnel: [w892] -> w879 mode=indexing
                            i -> [w897]
                            n257 = in-place {
                              in-place-border: w895 -> [w901]
                              in-place-border: [w899] -> w892
                              n258 = in-place-array #1(w898, w897) -> (w909:variant)
                              n259 = in-place-match #2(w894) -> (w906:errorcluster)
                              n260 = call <vilib>:"Get Type Information.vi"("error in (no error)"=w906, "variant"=w909) -> ("error out"=w905:errorcluster, "name"=w904:string)  [unwired: 5 in, 3 out]
                              n261 = call "LVJSON Find.vi"("Key"=w904, "Elements in"=w901) -> ("Found?"=w903:bool, "Index"=w902:i32)  [unwired: 8 in]
                              n262 = Index Array(array=w901, index=w902) -> (element=w900:T1)
                              n263 = case shown="True" w903 {
                                tunnel: w909 -> [w911 w912]
                                tunnel: [w911 w917] -> w908
                                tunnel: [w910 w916] -> w907
                                tunnel: w905 -> [w910 w915]
                                tunnel: w900 -> [_ w914]
                                tunnel: [_ w913] -> w899
                                frame False {
                                # "Key not\nfound,\nreturn type"
                                }
                                frame True {
                                # "Key\nFound"
                                n264 = call "LVJSON Unflatten.vi"("Variant Type"=w912, "error in (no error)"=w915, "Root Element in"=w914) -> ("error out"=w916:errorcluster, "Exists?"=w913:bool, "Variant out"=w917:variant)  [unwired: 5 in, 1 out]
                                }
                              }
                              n265 = in-place-array #1(w908) -> (w896:variant[])  [unwired: 1 out]
                              n266 = in-place-match #2(w907) -> (w893:errorcluster)
                            }
                          }
                          n267 = And Array Elements(Boolean array=w879) -> (logical AND=w884:bool)
                          n268 = call "Variant Cluster Create.vi"("error in (no error)"=w883, "Elements"=w881) -> ("error out"=w882:errorcluster, "Cluster"=w880:variant)  [unwired: 8 in]
                          n269 = call "Variant Preserve Type.vi"("Variant Type"=w889, "error in (no error)"=w882, "Variant in"=w880) -> ("error out"=w891:errorcluster, "Variant out"=w890:variant)  [unwired: 7 in]
                        }
                        frame True {
                          # "Is NULL element"
                        }
                      }
                    }
                    frame "Waveform" {
                      # "Return object as analog waveform"
                      n270 = Variant To Data(error in=w927, type=waveform(dbl) {"t0"=timestamp(0 s since 1904-01-01), "dt"=1.0, "Y"=[]} ("Waveform"), Variant=w926) -> (data=w936:waveform(dbl), error out=w928:errorcluster)
                      n271 = Unbundle By Name(w936) -> ("t0"=w942:timestamp, "dt"=w941:dbl, "Y"=w940:dbl[])
                      n272 = Bundle By Name(cluster=cluster{"t0":timestamp, "dt":dbl, "Y":dbl[]} {"t0"=timestamp(0 s since 1904-01-01), "dt"=0.0, "Y"=[]} ("Waveform"), "t0"=w942, "dt"=w941, "Y"=w940) -> (w937:cluster{"t0":timestamp, "dt":dbl, "Y":dbl[]})
                      n273 = To Variant(anything=w937) -> (Variant=w921:variant)
                      n274 = call "LVJSON Unflatten.vi"("Variant Type"=w921, "error in (no error)"=w928, "Root Element in"=w923) -> ("error out"=w939:errorcluster, "Exists?"=w922:bool, "Variant out"=w938:variant)  [unwired: 5 in, 1 out]
                      n275 = Variant To Data(error in=w939, type=w937, Variant=w938) -> (data=w935:cluster{"t0":timestamp, "dt":dbl, "Y":dbl[]}, error out=w925:errorcluster)
                      n276 = Unbundle By Name(w935) -> ("t0"=w932:timestamp, "dt"=w933:dbl, "Y"=w934:dbl[])
                      n277 = Bundle By Name(cluster=w936, "t0"=w932, "dt"=w933, "Y"=w934) -> (w931:waveform(dbl))
                      n278 = To Variant(anything=w931) -> (Variant=w924:variant)
                      n279 = call "Variant Preserve Type.vi"("Variant Type"=w926, "error in (no error)"=w925, "Variant in"=w924) -> ("error out"=w944:errorcluster, "Variant out"=w943:variant)  [unwired: 7 in]
                    }
                    frame "LV Variant" {
                      # "Return as\nVariant"
                      # "Return object as cluster variant"
                      n280 = for {
                        tunnel: w946 -> [w961] mode=indexing
                        shift-right: [w965] -> w953
                        shift-left: w947 -> [w962]
                        tunnel: [w963] -> w952 mode=indexing
                        tunnel: w945 -> [w959]
                        # "Set cluster element names"
                        n281 = call "LVJSON Unflatten.vi"("Variant Type"=w959, "error in (no error)"=w962, "Root Element in"=w961) -> ("error out"=w958:errorcluster, "Variant out"=w956:variant, "Key"=w960:string)  [unwired: 5 in, 1 out]
                        n282 = Variant To Data(error in=w958, type=variant, Variant=w956) -> (data=w955:variant, error out=w957:errorcluster)
                        n283 = call <vilib>:"Set Type Information.vi"("error in (no error)"=w957, "Name"=w960, "Variant in"=w955) -> ("error out"=w966:errorcluster, "Variant out"=w968:variant)  [unwired: 7 in]
                        n284 = Variant To Flattened String(Variant=w955) -> (data string=w964:string)  [unwired: 1 out]
                        n285 = Variant To Flattened String(Variant=w968) -> (1:w967:i16[])  [unwired: 1 out]
                        n286 = Flattened String To Variant(4:w966, 6:w964, 7:w967) -> (0:w965:errorcluster, 3:w963:variant)
                      }
                      n287 = call "Variant Cluster Create.vi"("error in (no error)"=w953, "Elements"=w952) -> ("error out"=w951:errorcluster, "Cluster"=w950:variant)  [unwired: 8 in]
                      n288 = To Variant(anything=w950) -> (Variant=w949:variant)
                    }
                    frame "Void" {
                      # "Return object as cluster variant"
                      n289 = for {
                        tunnel: w971 -> [w981] mode=indexing
                        shift-right: [w985] -> w976
                        shift-left: w972 -> [w982]
                        tunnel: [w983] -> w975 mode=indexing
                        tunnel: w970 -> [w979]
                        # "Set cluster element names"
                        n290 = call "LVJSON Unflatten.vi"("Variant Type"=w979, "error in (no error)"=w982, "Root Element in"=w981) -> ("error out"=w977:errorcluster, "Variant out"=w978:variant, "Key"=w980:string)  [unwired: 5 in, 1 out]
                        n291 = call <vilib>:"Set Type Information.vi"("error in (no error)"=w977, "Name"=w980, "Variant in"=w978) -> ("error out"=w986:errorcluster, "Variant out"=w988:variant)  [unwired: 7 in]
                        n292 = Variant To Flattened String(Variant=w978) -> (data string=w984:string)  [unwired: 1 out]
                        n293 = Variant To Flattened String(Variant=w988) -> (1:w987:i16[])  [unwired: 1 out]
                        n294 = Flattened String To Variant(4:w986, 6:w984, 7:w987) -> (0:w985:errorcluster, 3:w983:variant)
                      }
                      n295 = call "Variant Cluster Create.vi"("error in (no error)"=w976, "Elements"=w975) -> ("error out"=w974:errorcluster, "Cluster"=w969:variant)  [unwired: 8 in]
                    }
                  }
                }
                frame True {
                  n296 = To Variant(anything=w992) -> (Variant=w991:variant)
                }
              }
            }
          }
          n297 = case shown="Error .." w28 {
            selector: w28 -> [w993 w997]
            tunnel: [w993 w996] -> w31
            tunnel: w25 -> [_ w995]
            tunnel: w24 -> [_ w994]
            frame No Error {
            }
            frame Error {
              n298 = in-place {
                in-place-border: w995 -> [w999]
                in-place-border: w994 -> [w998]
                n299 = in-place-cluster #3(w997) -> ("source"=w1002:string)
                n300 = Format Into String(format string="\n\nLVJSON Type: %s\nKey: %s", initial string=w1002, w999, w998) -> (resulting string=w1001:string)  [unwired: 1 in, 1 out]
                n301 = in-place-cluster #3("source"=w1001) -> (w996:errorcluster)
              }
            }
          }
        }
      }
    }
    frame Error {
    }
  }
  "error out" <- w8
  "Variant out" <- w3
  "Key" <- w4
  "Exists?" <- w2
